vi "Clear Data.vi"(8 "error in (no error)":errorcluster, 11 "WebView2 Control in":refnum<class "WebView2 Control.lvclass">) -> (0 "error out":errorcluster, 3 "WebView2 Control out":refnum<class "WebView2 Control.lvclass">)   [LabVIEW 2020, in "WebView2.lvlib" / "WebView2 Control.lvclass"]
uses:
  WebView2 Control.lvclass
  C:/Users/Simon/Documents/GitHub/LV-WebView2/Source/Libs/Microsoft.Web.WebView2.Core.dll
  Libs/Microsoft.Web.WebView2.Core.dll
  Read Core.vi
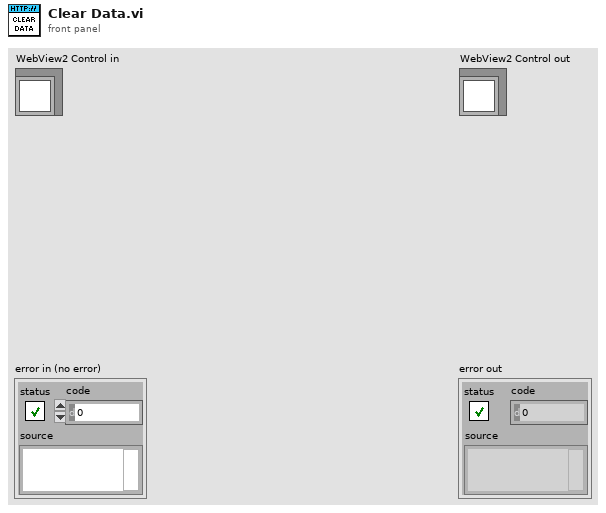
[diagram p1: front panel]
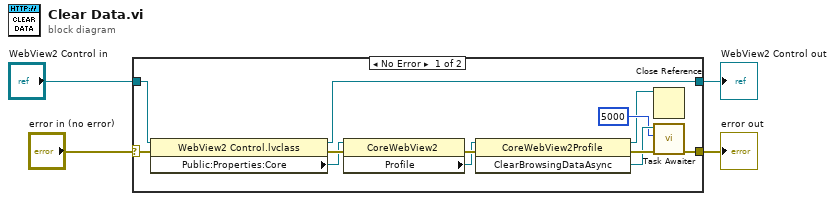
[diagram p0: block diagram]
diagram:
  n1 = case shown="No Error" "error in (no error)" {
    selector: "error in (no error)" -> [w16 w18]
    tunnel: [w8 w18] -> w3
    tunnel: [w13 w17] -> w1
    tunnel: "WebView2 Control in" -> [w14 w17]
    frame No Error {
      n2 = property class="WebView2 Control.lvclass"(reference=w14, error in=w16) -> (reference out=w13:refnum<class "WebView2 Control.lvclass">, error out=w15:errorcluster, "Public:Properties:Core"=w11:refnum<k24>)
      n3 = property class="CoreWebView2"(reference=w11, error in=w15) -> (error out=w12:errorcluster, "Profile"=w9:refnum<k24>)  [unwired: 1 out]
      n4 = invoke class="CoreWebView2Profile" method="ClearBrowsingDataAsync"(reference=w9, error in=w12) -> (reference out=w5:refnum<k24>, error out=w10:errorcluster, "ClearBrowsingDataAsync"=w7:refnum<k24>)  [unwired: 1 in]
      n5 = Close Reference(reference=w5) -> ()  [unwired: 1 in, 1 out]
      n6 = call "Task Awaiter.vi"("error in (no error)"=w10, "Timeout"=5000, "Task"=w7) -> ("error out"=w8:errorcluster)  [unwired: 6 in, 2 out]
    }
    frame Error {
    }
  }
  "error out" <- w3
  "WebView2 Control out" <- w1
